vi "Act 5.vi"() -> ()   [LabVIEW 2010]
uses:
  act/lv_01/lv_01.lvlib
panel:
  out "Deg F":dbl format="%.2f"
  out "Deg C":dbl format="%.2f"
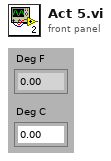
[diagram p1: front panel]
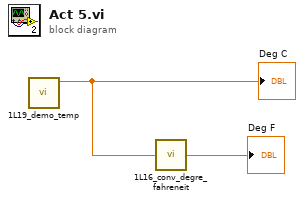
[diagram p0: block diagram]
diagram:
  n1 = call "1L19_demo_temp.vi"() -> ("temp"=w1:dbl)  [unwired: 6 in, 1 out]
  "Deg C" <- w1
  n2 = call "1L16_conv_degre_fahreneit.vi"("Deg C"=w1) -> ("Deg F"=→"Deg F":dbl)
